vi "Import Export - Temp SDF Dispose.vi"(8 "Error In":errorcluster, 10 "Temp SDF Path In":path, 11 "Temp SDF Refnum In":refnum<k24>) -> (0 "Error Out":errorcluster)   [LabVIEW 2017, in "Scan Engine Custom Device.lvlib"]
uses:
  Scan Engine Custom Device.lvlib
  NationalInstruments.VeriStand.SystemDefinitionAPI
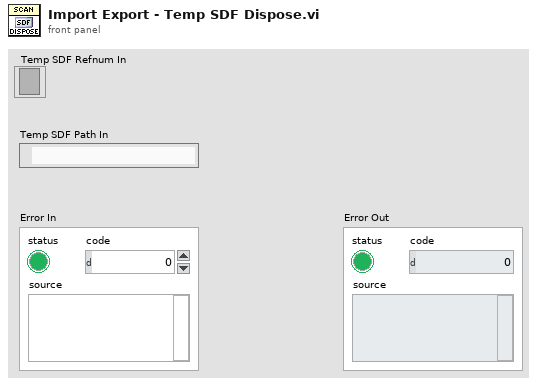
[diagram p1: front panel]
types:
  T1 = cluster{"Creator":string, "Target Name":string, "Target Type":string, "IP Address":string}
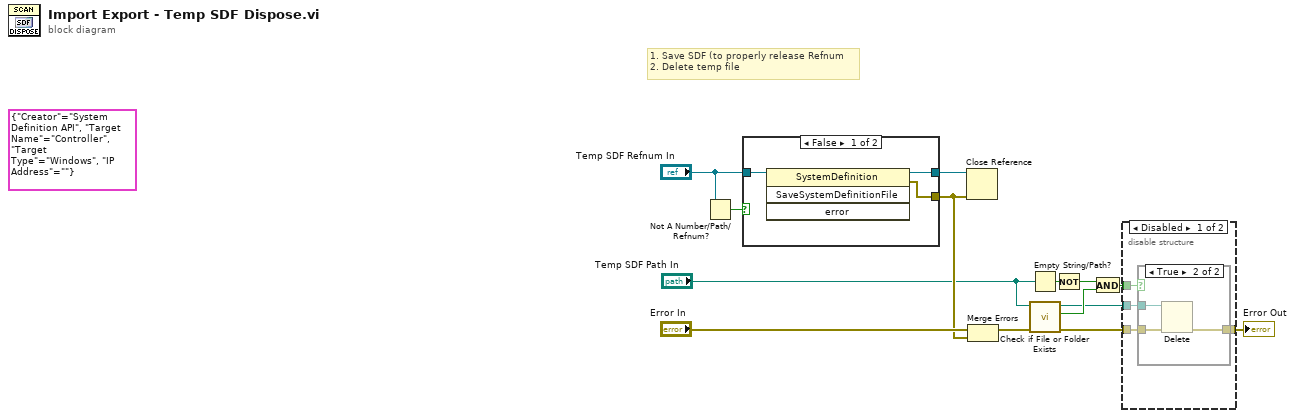
[diagram p0: block diagram]
diagram:
  (unwired) T1 {"Creator"="System Definition API", "Target Name"="Controller", "Target Type"="Windows", "IP Address"=""} ("New SDF Information")
  # "1. Save SDF (to properly release Refnum\n2. Delete temp file"
  n1 = Not A Number/Path/Refnum?(number/path/refnum="Temp SDF Refnum In") -> (NaN/Path/Refnum?=w11:bool)
  n2 = case shown="False" w11 {
    tunnel: [w17 w18] -> w14
    tunnel: "Temp SDF Refnum In" -> [w16 w18]
    tunnel: [w15 _] -> w10
    frame False {
      n3 = invoke class="SystemDefinition" method="SaveSystemDefinitionFile"(reference=w16) -> (reference out=w17:refnum<k24>, error out=w15:errorcluster)  [unwired: 3 in, 2 out]
    }
    frame True {
    }
  }
  n4 = Close Reference(reference=w14, error in (no error)=w10) -> ()  [unwired: 1 out]
  n5 = Merge Errors("Error In", w10) -> (w1:errorcluster)
  n6 = Empty String/Path?(string/path="Temp SDF Path In") -> (empty?=w8:bool)
  n7 = call <vilib>:"Check if File or Folder Exists.vi"("error in (no error)"=w1, "path"="Temp SDF Path In") -> ("error out"=w3:errorcluster, "file or folder exists?"=w7:bool, "dup path"=w4:path)  [unwired: 7 in]
  n8 = Not(x=w8) -> (.not. x?=w6:bool)
  n9 = And(x=w6, y=w7) -> (x .and. y?=w5:bool)
  n10 = disable-structure shown="Disabled" {
    disable-tunnel: w5 -> [w22 _]
    disable-tunnel: w4 -> [w21 _]
    disable-tunnel: w3 -> [w20 w27]
    disable-tunnel: [w19 w27] -> w2
    frame Disabled {
      n11 = case shown="True" w22 {
        tunnel: w21 -> [_ w26]
        tunnel: [w23 w25] -> w19
        tunnel: w20 -> [w23 w24]
        frame False {
        }
        frame True {
          n12 = Delete(path (use dialog)=w26, error in=w24) -> (error out=w25:errorcluster)  [unwired: 3 in, 2 out]
        }
      }
    }
    frame Enabled {
    }
  }
  "Error Out" <- w2
